vi "feedforward_3axis.vi"(0 "Xa1":dbl format="%#_13g", 1 "Ya1":dbl format="%#_13g", 2 "Za1":dbl format="%#_13g", 4 "w_jk_1":dbl format="%#_13g", 5 "w_x1":dbl format="%#_13g", 6 "w_x2":dbl format="%#_13g", 7 "w_x3":dbl format="%#_13g", 20 "w_y1":dbl format="%#_13g", 21 "w_y2":dbl format="%#_13g", 22 "w_y3":dbl format="%#_13g", 23 "w_jk_2":dbl format="%#_13g", 24 "w_jk_3":dbl format="%#_13g", 25 "w_z1":dbl format="%#_13g", 26 "w_z2":dbl format="%#_13g", 27 "w_z3":dbl format="%#_13g") -> (9 "x_j":dbl, 11 "x_k":dbl, 16 "z_j":dbl, 17 "y_j":dbl, 18 "z_k":dbl, 19 "y_k":dbl)   [LabVIEW 2014]
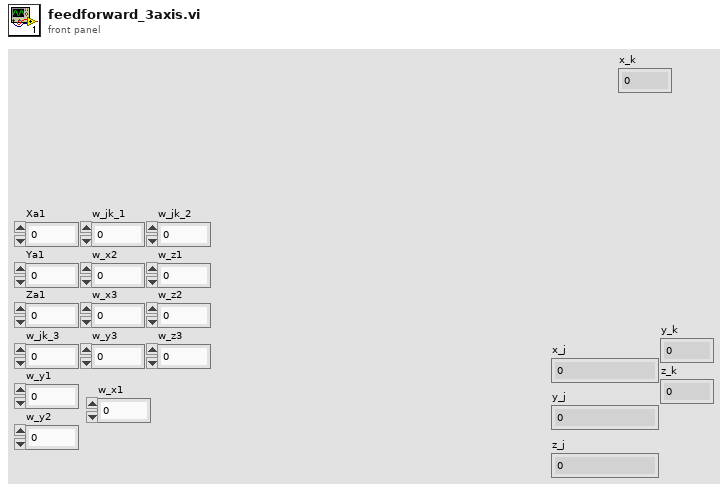
[diagram p1: front panel]
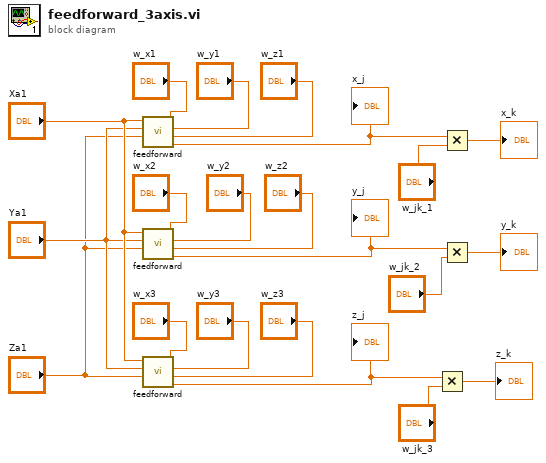
[diagram p0: block diagram]
diagram:
  n1 = call "feedforward.vi"("Zmult"="w_z1", "Ymult"="w_y1", "Xmult"="w_x1", "Zacc"="Za1", "Yacc"="Ya1", "Xacc"="Xa1") -> ("Output (0to1)"=w1:dbl)  [unwired: 5 in]
  "x_j" <- w1
  n2 = call "feedforward.vi"("Zmult"="w_z2", "Ymult"="w_y2", "Xmult"="w_x2", "Zacc"="Za1", "Yacc"="Ya1", "Xacc"="Xa1") -> ("Output (0to1)"=w2:dbl)  [unwired: 5 in]
  "y_j" <- w2
  n3 = call "feedforward.vi"("Zmult"="w_z3", "Ymult"="w_y3", "Xmult"="w_x3", "Zacc"="Za1", "Yacc"="Ya1", "Xacc"="Xa1") -> ("Output (0to1)"=w3:dbl)  [unwired: 5 in]
  "z_j" <- w3
  n4 = Multiply(x=w3, y="w_jk_3") -> (x*y=→"z_k":dbl)
  n5 = Multiply(x=w1, y="w_jk_1") -> (x*y=→"x_k":dbl)
  n6 = Multiply(x=w2, y="w_jk_2") -> (x*y=→"y_k":dbl)
